vi "To Gray_FPGA (SubVI).vi"(10 "Pixel Data":cluster{"A":u8, "R/H":u8, "G/S":u8, "B/L":u8}) -> (2 "Data Out":fxp<+,8,8>)   [LabVIEW 2016]
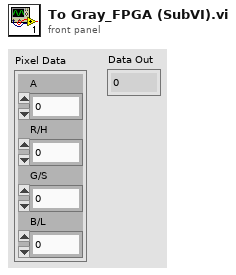
[diagram p1: front panel]
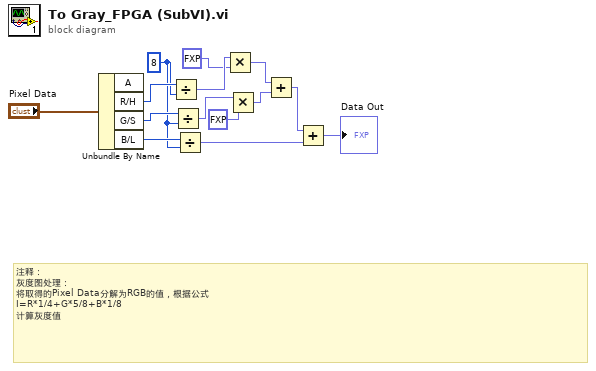
[diagram p0: block diagram]
diagram:
  w10 = u8 8 ("y")
  # "注释：\n灰度图处理：\n将取得的Pixel Data分解为RGB的值，根据公式\nI=R*1/4+G*5/8+B*1/8\n计算灰度值"
  n1 = Unbundle By Name("Pixel Data") -> ("R/H"=w13:u8, "G/S"=w12:u8, "B/L"=w11:u8)  [unwired: 1 out]
  n2 = Divide(x=w13, y=w10) -> (x/y=w9:fxp<+,5,5>)
  n3 = Divide(x=w12, y=w10) -> (x/y=w7:fxp<+,5,5>)
  n4 = Divide(x=w11, y=w10) -> (x/y=w2:fxp<+,5,5>)
  n5 = Multiply(x=w9, y=fxp<+/-,32,26> 2.0) -> (x*y=w5:fxp<+,6,6>)
  n6 = Multiply(x=w7, y=fxp<+/-,32,26> 5.0) -> (x*y=w4:fxp<+,8,8>)
  n7 = Add(x=w5, y=w4) -> (x+y=w3:fxp<+,8,8>)
  n8 = Add(x=w3, y=w2) -> (x+y=→"Data Out":fxp<+,8,8>)
